vi "密码输入窗口.vi"(11 "权限等级":i32) -> (3 "结果":bool)   [LabVIEW 2018]
panel:
  out "取消按钮":bool
  out "确定登录":bool
  in  "字符串":string
  in  "下拉列表":u16(ring) items=["user1", "user2", "user3", "user4", "user5"]
  # "用户权限登录"
  # "用户"
  # "密码"
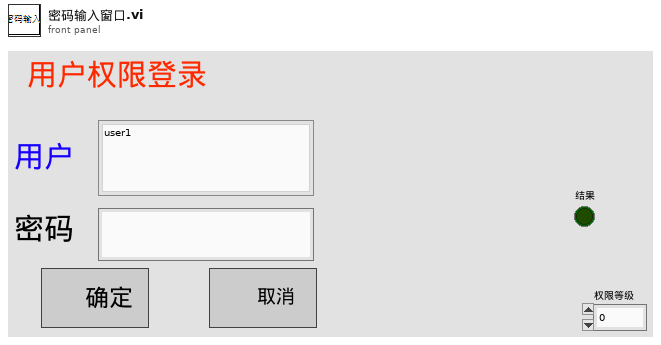
[diagram p1: front panel]
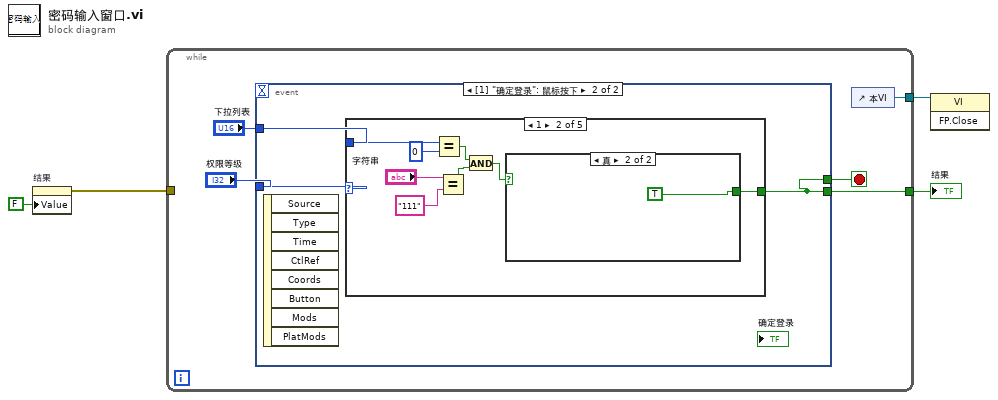
[diagram p0: block diagram]
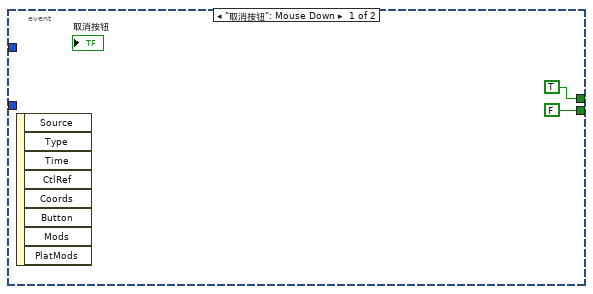
[diagram p2: hidden frame]
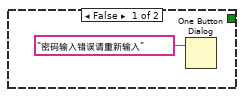
[diagram p4: hidden frame]
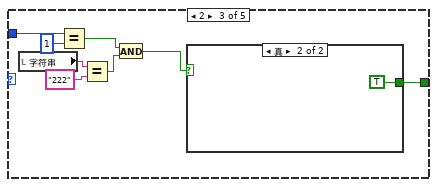
[diagram p5: hidden frame]
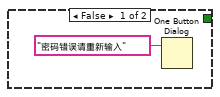
[diagram p6: hidden frame]
diagram:
  n1 = property on="结果" class="Bool (严格)"("Value"=FALSE ("结果")) -> (error out=w2:errorcluster)  [unwired: 2 in, 1 out]
  n2 = while {
    tunnel: [w9] -> w4
    tunnel: [w5] -> w3
    tunnel: w2 -> [_]
    stop <- w8 stop-if-true
    n3 = event shown="[1] \"确定登录\": 鼠标按下" {
      selector: _ -> [_ _]
      dyn-events: _ -> [_ _]
      timeout: _ -> [_ _]
      tunnel: [FALSE w12] -> w9
      tunnel: [TRUE w12] -> w8
      tunnel: "权限等级" -> [_ w14]
      tunnel: "下拉列表" -> [_ w13]
      event "取消按钮": Mouse Down {
        n4 = event-data() -> ()  [unwired: 1 in, 8 out]
      }
      event "确定登录": Mouse Down {
        n5 = event-data() -> ()  [unwired: 1 in, 8 out]
        n6 = case shown="1" w14 {
          tunnel: w13 -> [_ w20 w30 _ _]
          tunnel: [_ w21 w31 _ _] -> w12
          frame 0, Default {
          }
          frame 1 {
            n7 = Equal?(x=w20, y=u16 0) -> (x = y?=w18:bool)
            n8 = Equal?(x="字符串", y="111") -> (x = y?=w17:bool)
            n9 = And(x=w18, y=w17) -> (x .and. y?=w16:bool)
            n10 = case shown="真" w16 {
              tunnel: [_ TRUE] -> w21
              frame False {
                n11 = One Button Dialog(message="密码输入错误请重新输入" ("消息")) -> ()  [unwired: 1 in, 1 out]
              }
              frame True {
              }
            }
          }
          frame 2 {
            n12 = local read "字符串"() -> (w25:string)
            n13 = Equal?(x=w30, y=u16 1) -> (x = y?=w28:bool)
            n14 = Equal?(x=w25, y="222") -> (x = y?=w27:bool)
            n15 = And(x=w28, y=w27) -> (x .and. y?=w26:bool)
            n16 = case shown="真" w26 {
              tunnel: [_ TRUE] -> w31
              frame False {
                n17 = One Button Dialog(message="密码错误请重新输入" ("消息")) -> ()  [unwired: 1 in, 1 out]
              }
              frame True {
              }
            }
          }
          frame 3 {
          }
          frame 4 {
          }
        }
      }
    }
    n18 = control-ref of="本VI"() -> (w5:refnum<vi>)
  }
  "结果" <- w4
  n19 = invoke class="VI" method="FP.Close"(reference=w3) -> ()  [unwired: 2 in, 3 out]
